vi "AI Channel Read.vi"(8 "error in":errorcluster, 10 "input terminal configuration":i32(ring)=10078 items=["default"=-1, "RSE"=10083, "NRSE"=10078, "Differential"=10106, "Pseudodifferential"=12529], 11 "physical channels":tag) -> (0 "error out":errorcluster, 3 "data":dbl format="%.4f")   [LabVIEW 2015]
uses:
  <vilib>/DAQmx/read.llb/DAQmx Read (Analog DBL 1Chan 1Samp).vi
  <vilib>/DAQmx/create/channels.llb/DAQmx Create Channel (AI-Voltage-Basic).vi
  <vilib>/DAQmx/miscellaneous.llb/DAQmx Fill In Error Info.vi
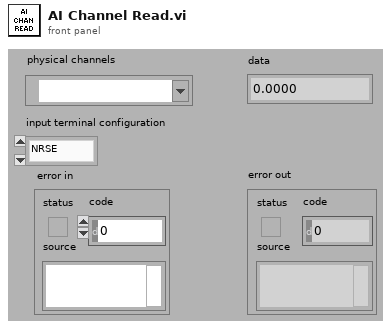
[diagram p1: front panel]
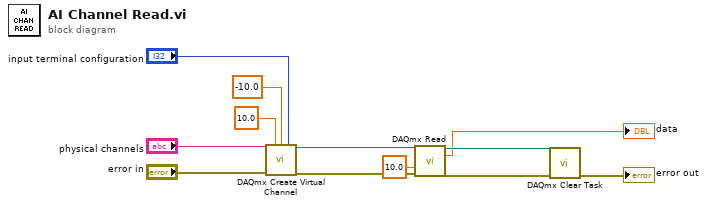
[diagram p0: block diagram]
diagram:
  n1 = call-poly <vilib>:"DAQmx Create Virtual Channel.vi"("maximum value"=10.0, "minimum value"=-10.0, "input terminal configuration"="input terminal configuration", "physical channels"="physical channels", "error in"="error in") -> ("task out"=w7:refnum<k21>, "error out"=w8:errorcluster)  [unwired: 9 in]
  n2 = call-poly <vilib>:"DAQmx Read.vi"("task/channels in"=w7, "timeout"=10.0, "error in"=w8) -> ("task out"=w4:refnum<k21>, "data"=→"data":dbl, "error out"=w5:errorcluster)  [unwired: 10 in]
  n3 = call <vilib>:"DAQmx Clear Task.vi"("task in"=w4, "error in"=w5) -> ("error out"=→"error out":errorcluster)  [unwired: 13 in]
